vi "test_HostApi TimeOut Error.vi"(8 "error in (no error)":errorcluster) -> (0 "error out":errorcluster)   [LabVIEW 2019, in "Host API Tests.lvclass"]
uses:
  Host API Tests.lvclass
  Addon/Addon Shared/Types/Buffered RT Instrument Command.ctl
  Addon/Addon Shared/Types/Response Wait Type.ctl
  <vilib>/addons/_JKI Toolkits/VI Tester/TestCase.llb/TestCase.lvclass
  APIs/Host Automation API/Instrument Host Automation API.lvlib
  Addon/Addon Shared/Instrument Addon Shared.lvlib
  C:/Program Files (x86)/National Instruments/LabVIEW 2019/vi.lib/addons/_JKI Toolkits/VI Tester/TestCase.llb/TestCase.lvclass
panel:
  out "TestCase out":refnum<class "Host API Tests.lvclass">
  in  "TestCase in":refnum<class "Host API Tests.lvclass">
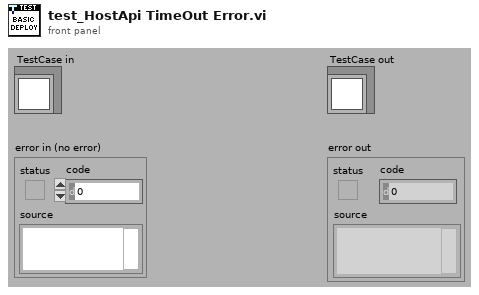
[diagram p1: front panel]
types:
  T1 = typedef "Instrument Addon Shared.lvlib/Buffered RT Instrument Command.ctl" = cluster{"Command":string, "Response Expected?":bool, "Wait Type":T2, "Wait Value":dbl}
  T2 = typedef "Instrument Addon Shared.lvlib/Response Wait Type.ctl" = enum16{"Byte Count", "Wait sec"}
  T3 = typedef "NI STM.lvlib/TCP Connection Info.ctl" = cluster{"connection ID":refnum<k5>, "meta data":T4[]}
  T4 = typedef "NI STM.lvlib/MetaDataElement.ctl" = string
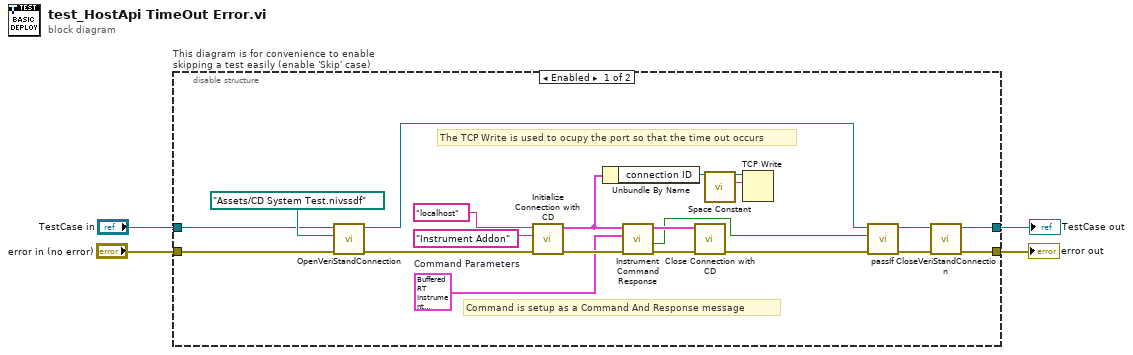
[diagram p0: block diagram]
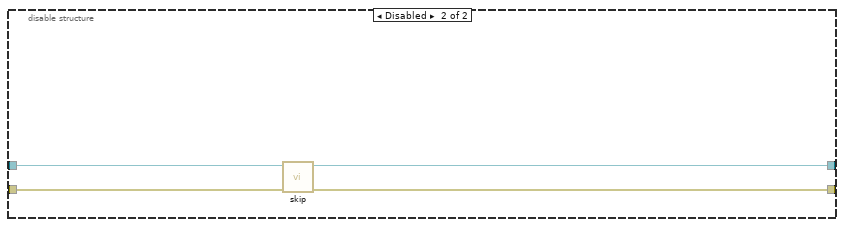
[diagram p2: hidden frame]
diagram:
  n1 = disable-structure "This diagram is for convenience to enable skipping a test easily (enable 'Skip' case)" shown="Enabled" {
    disable-tunnel: "TestCase in" -> [w20 w28]
    disable-tunnel: [w18 w26] -> w1
    disable-tunnel: [w19 w27] -> w3
    disable-tunnel: "error in (no error)" -> [w21 w25]
    frame Enabled {
      w5 = T1 {"Command"="15CommandResponse", "Response Expected?"=TRUE, "Wait Type"=enum."Byte Count", "Wait Value"=17.0}  # Command Parameters
      # "The TCP Write is used to ocupy the port so that the time out occurs"
      # "Command is setup as a Command And Response message"
      n2 = call-dynamic "OpenVeriStandConnection.vi"("error in (no error)"=w21, "System Definition File"=path "Assets/CD System Test.nivssdf", "VeriStand Test Case in"=w20) -> ("error out"=w17:errorcluster, "VeriStand Test Case out"=w10:refnum<class "Host API Tests.lvclass">)  [unwired: 6 in, 1 out]
      n3 = call "Initialize Connection with CD.vi"("error in (no error)"=w17, "TCP Service"="Instrument Addon", "IP Address"="localhost") -> ("error out"=w14:errorcluster, "connection info out"=w9:T3)  [unwired: 7 in]
      n4 = Unbundle By Name(w9) -> ("connection ID"=w8:refnum<k5>)
      n5 = call "Instrument Command Response.vi"("error in (no error)"=w14, "Command Parameters"=w5, "Comm.Info"=w9) -> ("error out"=w12:errorcluster, "Timed Out?"=w7:bool, "Comm.Info"=w11:T3)  [unwired: 5 in, 1 out]
      n6 = call "Close Connection with CD.vi"("error in"=w12, "Comm.Info"=w11) -> ("error out"=w13:errorcluster)  [unwired: 9 in]
      n7 = call <vilib>:"Space Constant.vi"() -> ("String"=w6:string)
      n8 = TCP Write(connection ID=w8, data in=w6) -> ()  [unwired: 2 in, 3 out]
      n9 = call-dynamic "passIf.vi"("error in (no error)"=w13, "pass"=w7, "TestCase in"=w10) -> ("error out"=w16:errorcluster, "TestCase out"=w15:refnum<class "Host API Tests.lvclass">)  [unwired: 7 in]
      n10 = call-dynamic "CloseVeriStandConnection.vi"("error in (no error)"=w16, "VeriStand Test Case in"=w15) -> ("error out"=w19:errorcluster, "VeriStand Test Case out"=w18:refnum<class "Host API Tests.lvclass">)  [unwired: 8 in]
    }
    frame Disabled {
      # "skip test result while test is under development"
      n11 = call <vilib>:"skip.vi"("error in (no error)"=w25, "TestCase in"=w28) -> ("error out"=w27:errorcluster, "TestCase out"=w26:refnum<class "Host API Tests.lvclass">)  [unwired: 8 in]
    }
  }
  "error out" <- w3
  "TestCase out" <- w1
